vi "Read Coordinates T+1.vi"(11 "Movable in":refnum<class "Movable.lvclass">) -> (2 "Coordinates":T1)   [LabVIEW 2021, in "Movable.lvclass"]
doc: "MIT Licence\nCopyright (c) 2024 David Grollier"
uses:
  Movable.lvclass
  Type Def/Coordinates.ctl
  Movable.lvclass/Movable.ctl
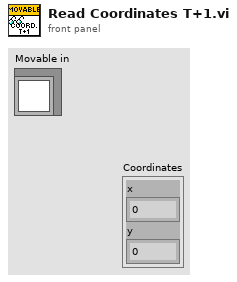
[diagram p1: front panel]
types:
  T1 = typedef "Coordinates.ctl" = cluster{"x":dbl, "y":dbl}
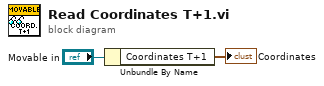
[diagram p0: block diagram]
diagram:
  n1 = Unbundle By Name("Movable in") -> ("Coordinates T+1"=→"Coordinates":T1)
